vi "Subscribe.vi"(8 "error in (no error)":errorcluster, 10 "SubscriptionRequest":refnum<class "SubscriptionRequest.lvclass">, 11 "IController in":refnum<class "IController.lvclass">) -> (0 "error out":errorcluster, 3 "IController out":refnum<class "IController.lvclass">)   [LabVIEW 2015, in "IController.lvlib" / "IController.lvclass"]
uses:
  IController.lvclass
  IMediator/SubscriptionRequest/SubscriptionRequest.lvclass
  IController.lvclass/IController.ctl
  IMediator/IMediator Messages/Subscribe Msg/Subscribe Msg.lvclass/Subscribe Msg.ctl
  <vilib>/ActorFramework/Message Enqueuer/Message Enqueuer.lvclass/Message Enqueuer.ctl
  <vilib>/ActorFramework/Message Enqueuer/Enqueue.vi
  <vilib>/ActorFramework/Message Priority Queue/Priority Enqueue.vi
  IMediator/IMediator Messages/Subscribe Msg/Subscribe Msg.lvclass
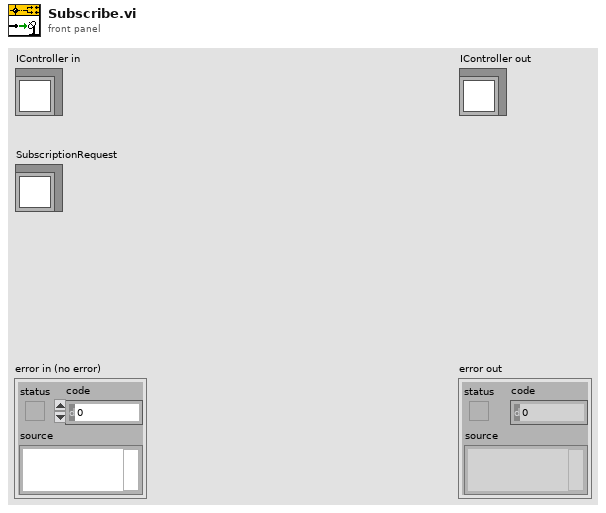
[diagram p1: front panel]
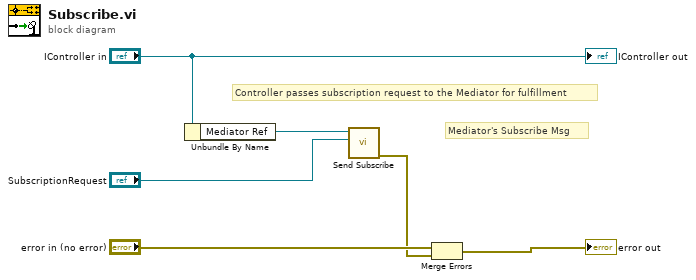
[diagram p0: block diagram]
diagram:
  # "Mediator's Subscribe Msg"
  # "Controller passes subscription request to the Mediator for fulfillment"
  n1 = Unbundle By Name("IController in") -> ("Mediator Ref"=w4:refnum<class "Message Enqueuer.lvclass">)
  n2 = call "Send Subscribe.vi"("Subscription Request"="SubscriptionRequest", "Message Enqueuer"=w4) -> ("error out"=w1:errorcluster)  [unwired: 8 in, 1 out]
  n3 = Merge Errors("error in (no error)", w1) -> (→"error out":errorcluster)
  "IController out" <- "IController in"
